vi "Control_SR830.vi"() -> ()   [LabVIEW 2015]
panel:
  in  "GPIB Address":string="1"
  in  "Record new values":bool
  out "Y (V)":dbl
  out "X (V)":dbl
  out "Harmonic #":dbl
  out "Phase":dbl
  out "Oscillator (V)":dbl
  out "Frequency (Hz)":dbl
  out "Time Constant":u16(ring) items=["10 us", "30 us", "100 us", "300 us", "1 ms", "3 ms", "10 ms", "30 ms", "100 ms", "300 ms", "1 s", "3 s", "10 s", "30 s", "100 s", "300 s", "1 ks", "3 ks", "10 ks", "30 ks"]
  out "Sensitivity":u16(ring) items=["2 nV", "5 nV", "10 nV", "20 nV", "50 nV", "100 nV", "200 nV", "500 nV", "1 uV", "2 uV", "5 uV", "10 uV", "20 uV", "50 uV", "100 uV", "200 uV", "500 uV", "1 mV", "2 mV", "5 mV", "10 mV", "20 mV", "50 mV", "100 mV", "200 mV", "500 mV", "1 V"]
  in  "ON/OFF channel":bool
  in  "error in (no error)":errorcluster
  out "error out":errorcluster
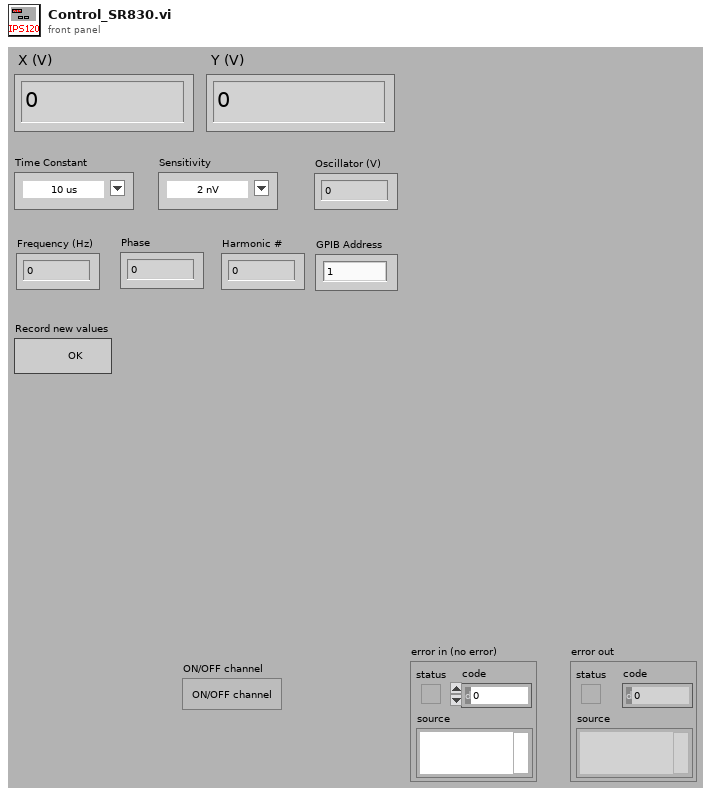
[diagram p1: front panel]
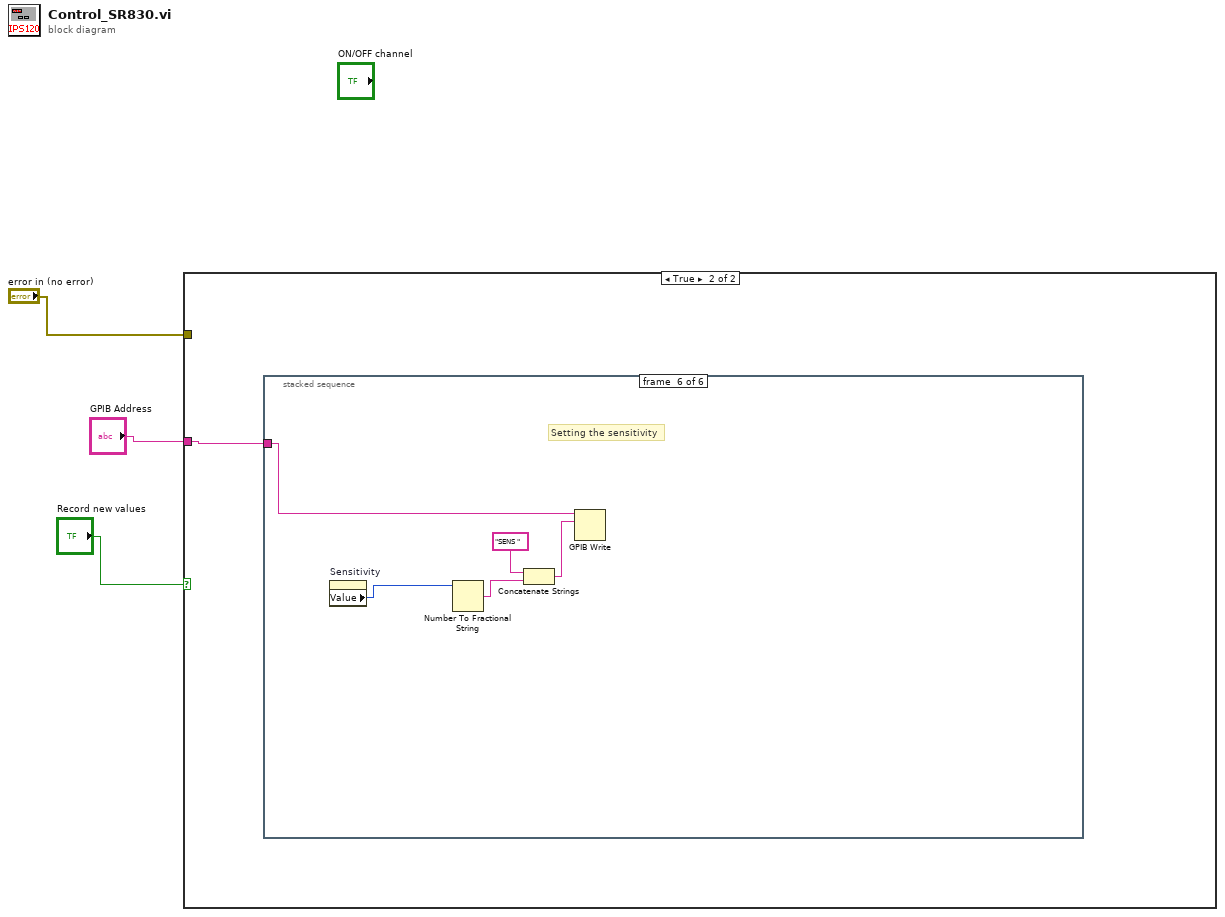
[diagram p0: block diagram]
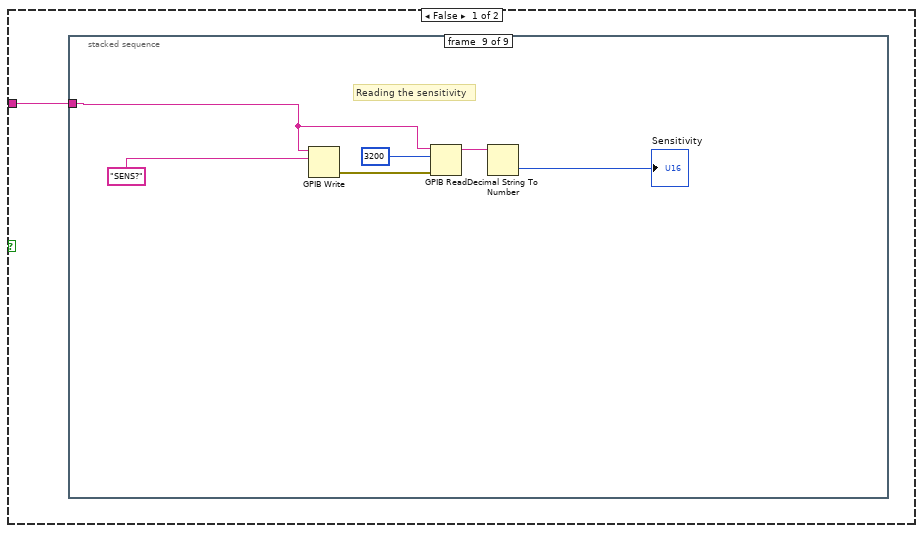
[diagram p2: hidden frame]
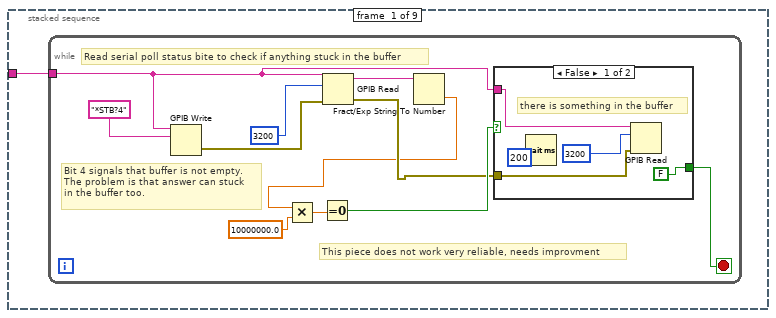
[diagram p3: hidden frame]
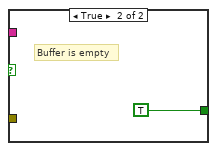
[diagram p4: hidden frame]
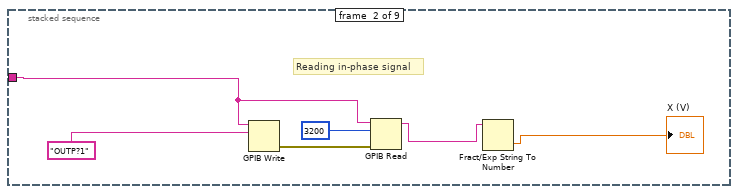
[diagram p5: hidden frame]
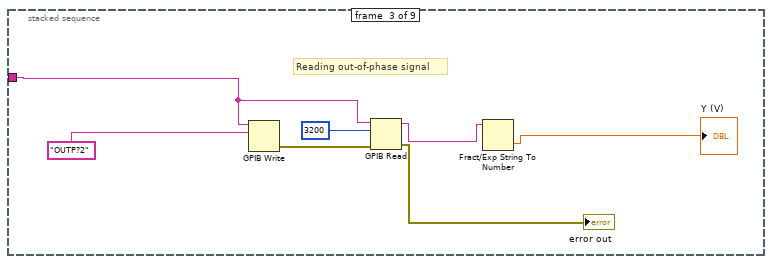
[diagram p6: hidden frame]
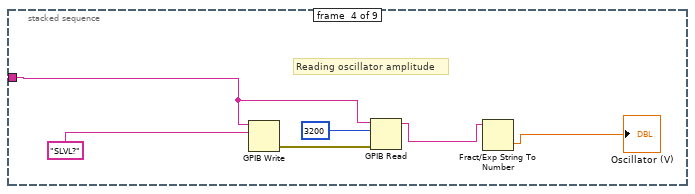
[diagram p7: hidden frame]
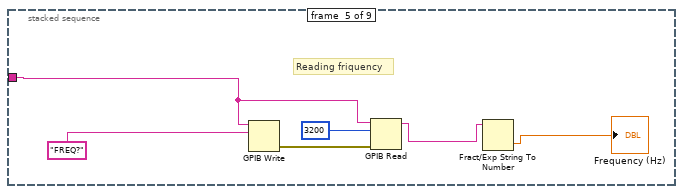
[diagram p8: hidden frame]
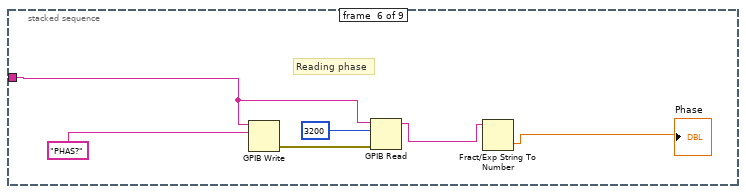
[diagram p9: hidden frame]
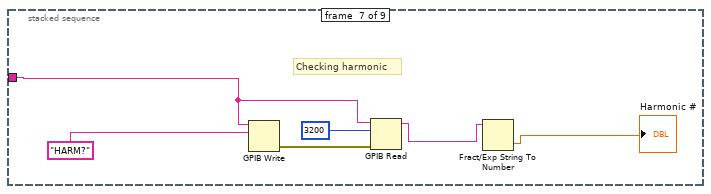
[diagram p10: hidden frame]
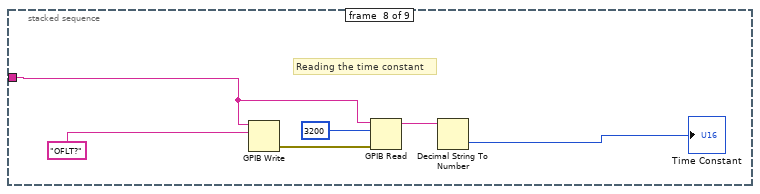
[diagram p11: hidden frame]
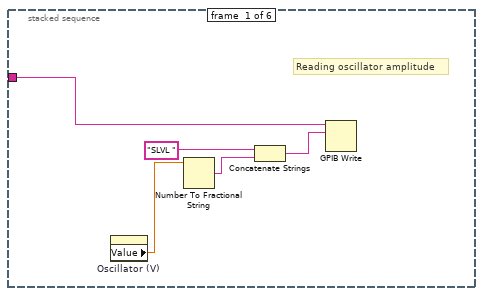
[diagram p12: hidden frame]
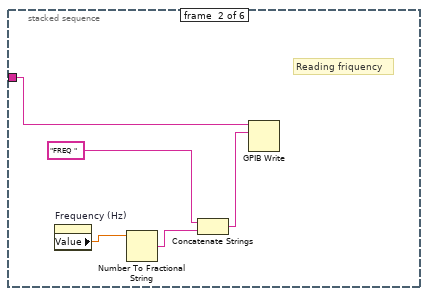
[diagram p13: hidden frame]
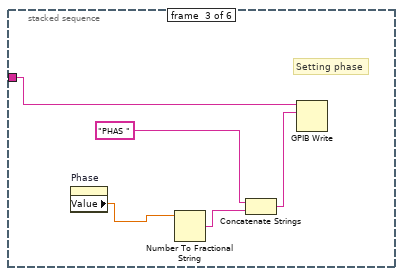
[diagram p14: hidden frame]
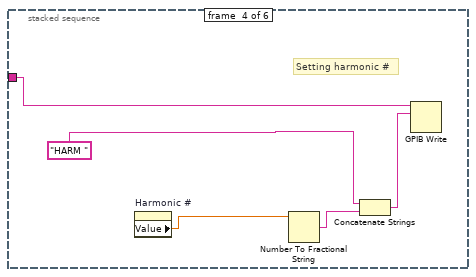
[diagram p15: hidden frame]
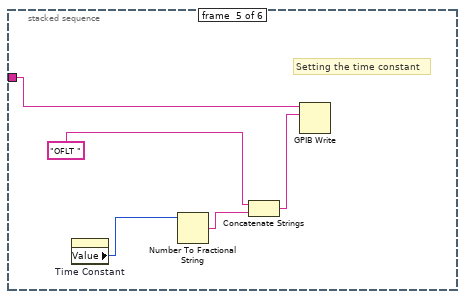
[diagram p16: hidden frame]
diagram:
  n1 = case shown="True" "Record new values" {
    tunnel: "GPIB Address" -> [w4 w72]
    tunnel: "error in (no error)" -> [_ _]
    frame False {
      n2 = stacked-sequence {
        tunnel: w4 -> [w5 w23 w30 w36 w42 w48 w54 w60 w66]
        frame #0 {
          n3 = while {
            tunnel: w5 -> [w12]
            stop <- w11 stop-if-true
            # "Bit 4 signals that buffer is not empty.\nThe problem is that answer can stuck\nin the buffer too."
            # "Read serial poll status bite to check if anything stuck in the buffer"
            # "This piece does not work very reliable, needs improvment"
            n4 = GPIB Write(0:w12, 1:"*STB?4") -> (6:w15:errorcluster)  [unwired: 3 in, 1 out]
            n5 = GPIB Read(0:w12, 1:3200, 3:w15) -> (5:w13:string, 7:w9:errorcluster)  [unwired: 2 in, 1 out]
            n6 = Fract/Exp String To Number(string=w13) -> (number=w7:dbl)  [unwired: 3 in, 1 out]
            n7 = Multiply(x=w7, y=10000000.0) -> (x*y=w8:dbl)
            n8 = Equal To 0?(x=w8) -> (x = 0?=w10:bool)
            n9 = case shown="False" w10 {
              tunnel: w12 -> [w20 _]
              tunnel: [FALSE TRUE] -> w11
              tunnel: w9 -> [w18 _]
              frame False {
                # "there is something in the buffer"
                n10 = Wait (ms)(milliseconds to wait=200) -> ()  [unwired: 1 out]
                n11 = GPIB Read(0:w20, 1:3200, 3:w18) -> ()  [unwired: 2 in, 3 out]
              }
              frame True {
                # "Buffer is empty"
              }
            }
          }
        }
        frame #1 {
          # "Reading in-phase signal"
          n12 = GPIB Write(0:w23, 1:"OUTP?1") -> (6:w28:errorcluster)  [unwired: 3 in, 1 out]
          n13 = GPIB Read(0:w23, 1:3200, 3:w28) -> (5:w25:string)  [unwired: 2 in, 2 out]
          n14 = Fract/Exp String To Number(string=w25) -> (number=→"X (V)":dbl)  [unwired: 3 in, 1 out]
        }
        frame #2 {
          # "Reading out-of-phase signal"
          n15 = GPIB Write(0:w30, 1:"OUTP?2") -> (6:w35:errorcluster)  [unwired: 3 in, 1 out]
          n16 = GPIB Read(0:w30, 1:3200, 3:w35) -> (5:w32:string, 7:→"error out":errorcluster)  [unwired: 2 in, 1 out]
          n17 = Fract/Exp String To Number(string=w32) -> (number=→"Y (V)":dbl)  [unwired: 3 in, 1 out]
        }
        frame #3 {
          # "Reading oscillator amplitude"
          n18 = GPIB Write(0:w36, 1:"SLVL?") -> (6:w41:errorcluster)  [unwired: 3 in, 1 out]
          n19 = GPIB Read(0:w36, 1:3200, 3:w41) -> (5:w38:string)  [unwired: 2 in, 2 out]
          n20 = Fract/Exp String To Number(string=w38) -> (number=→"Oscillator (V)":dbl)  [unwired: 3 in, 1 out]
        }
        frame #4 {
          # "Reading friquency"
          n21 = GPIB Write(0:w42, 1:"FREQ?") -> (6:w47:errorcluster)  [unwired: 3 in, 1 out]
          n22 = GPIB Read(0:w42, 1:3200, 3:w47) -> (5:w44:string)  [unwired: 2 in, 2 out]
          n23 = Fract/Exp String To Number(string=w44) -> (number=→"Frequency (Hz)":dbl)  [unwired: 3 in, 1 out]
        }
        frame #5 {
          # "Reading phase"
          n24 = GPIB Write(0:w48, 1:"PHAS?") -> (6:w53:errorcluster)  [unwired: 3 in, 1 out]
          n25 = GPIB Read(0:w48, 1:3200, 3:w53) -> (5:w50:string)  [unwired: 2 in, 2 out]
          n26 = Fract/Exp String To Number(string=w50) -> (number=→"Phase":dbl)  [unwired: 3 in, 1 out]
        }
        frame #6 {
          # "Checking harmonic"
          n27 = GPIB Write(0:w54, 1:"HARM?") -> (6:w59:errorcluster)  [unwired: 3 in, 1 out]
          n28 = GPIB Read(0:w54, 1:3200, 3:w59) -> (5:w56:string)  [unwired: 2 in, 2 out]
          n29 = Fract/Exp String To Number(string=w56) -> (number=→"Harmonic #":dbl)  [unwired: 3 in, 1 out]
        }
        frame #7 {
          # "Reading the time constant"
          n30 = GPIB Write(0:w60, 1:"OFLT?") -> (6:w65:errorcluster)  [unwired: 3 in, 1 out]
          n31 = GPIB Read(0:w60, 1:3200, 3:w65) -> (5:w62:string)  [unwired: 2 in, 2 out]
          n32 = Decimal String To Number(string=w62) -> (number=→"Time Constant":i32)  [unwired: 2 in, 1 out]
        }
        frame #8 {
          # "Reading the sensitivity"
          n33 = GPIB Write(0:w66, 1:"SENS?") -> (6:w71:errorcluster)  [unwired: 3 in, 1 out]
          n34 = GPIB Read(0:w66, 1:3200, 3:w71) -> (5:w68:string)  [unwired: 2 in, 2 out]
          n35 = Decimal String To Number(string=w68) -> (number=→"Sensitivity":i32)  [unwired: 2 in, 1 out]
        }
      }
    }
    frame True {
      n36 = stacked-sequence {
        tunnel: w72 -> [w73 w78 w84 w88 w93 w98]
        frame #0 {
          # "Reading oscillator amplitude"
          n37 = property on="Oscillator (V)" class="DigNum (strict)"() -> ("Value"=w77:dbl)  [unwired: 2 in, 2 out]
          n38 = Number To Fractional String(number=w77) -> (F-format string=w76:string)  [unwired: 3 in]
          n39 = Concatenate Strings("SLVL ", w76) -> (w75:string)
          n40 = GPIB Write(0:w73, 1:w75) -> ()  [unwired: 3 in, 2 out]
        }
        frame #1 {
          # "Reading friquency"
          n41 = property on="Frequency (Hz)" class="DigNum (strict)"() -> ("Value"=w80:dbl)  [unwired: 2 in, 2 out]
          n42 = Number To Fractional String(number=w80) -> (F-format string=w82:string)  [unwired: 3 in]
          n43 = Concatenate Strings("FREQ ", w82) -> (w79:string)
          n44 = GPIB Write(0:w78, 1:w79) -> ()  [unwired: 3 in, 2 out]
        }
        frame #2 {
          # "Setting phase"
          n45 = property on="Phase" class="DigNum (strict)"() -> ("Value"=w83:dbl)  [unwired: 2 in, 2 out]
          n46 = Number To Fractional String(number=w83) -> (F-format string=w87:string)  [unwired: 3 in]
          n47 = Concatenate Strings("PHAS ", w87) -> (w85:string)
          n48 = GPIB Write(0:w84, 1:w85) -> ()  [unwired: 3 in, 2 out]
        }
        frame #3 {
          # "Setting harmonic #"
          n49 = property on="Harmonic #" class="DigNum (strict)"() -> ("Value"=w89:dbl)  [unwired: 2 in, 2 out]
          n50 = Number To Fractional String(number=w89) -> (F-format string=w92:string)  [unwired: 3 in]
          n51 = Concatenate Strings("HARM ", w92) -> (w91:string)
          n52 = GPIB Write(0:w88, 1:w91) -> ()  [unwired: 3 in, 2 out]
        }
        frame #4 {
          # "Setting the time constant"
          n53 = property on="Time Constant" class="Ring (strict)"() -> ("Value"=w94:u16)  [unwired: 2 in, 2 out]
          n54 = Number To Fractional String(number=w94) -> (F-format string=w97:string)  [unwired: 3 in]
          n55 = Concatenate Strings("OFLT ", w97) -> (w96:string)
          n56 = GPIB Write(0:w93, 1:w96) -> ()  [unwired: 3 in, 2 out]
        }
        frame #5 {
          # "Setting the sensitivity"
          n57 = property on="Sensitivity" class="Ring (strict)"() -> ("Value"=w99:u16)  [unwired: 2 in, 2 out]
          n58 = Number To Fractional String(number=w99) -> (F-format string=w102:string)  [unwired: 3 in]
          n59 = Concatenate Strings("SENS ", w102) -> (w101:string)
          n60 = GPIB Write(0:w98, 1:w101) -> ()  [unwired: 3 in, 2 out]
        }
      }
    }
  }
